vi "State.vi"(8 "error in (no error)":errorcluster caption="entrée d'erreur (pas d'erreur)", 10 "State":T1(ring), 11 "Actor_EventStart en entrée":refnum<class "Actor_EventStart.lvclass">) -> (0 "error out":errorcluster caption="sortie d'erreur", 3 "Actor_EventStart en sortie":refnum<class "Actor_EventStart.lvclass">)   [LabVIEW 2020, in "Library Core.lvlib" / "Actor_EventStart.lvlib" / "Actor_EventStart.lvclass"]
uses:
  Actor_EventStart.lvclass
  Commun VI/TypeDef/Variable Printable.ctl
  Actor_EventStart.lvclass/Actor_EventStart.ctl
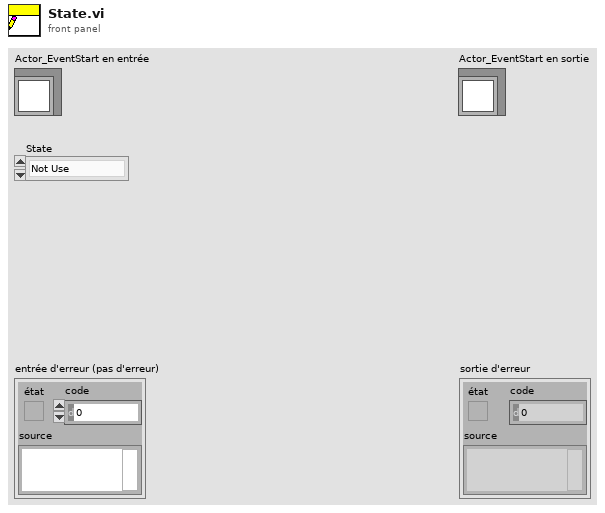
[diagram p1: front panel]
types:
  T1 = enum16{"Not Use", "Wait Event", "Test in progress", "Test Stopped"}
  T2 = enum16{"Get Variable", "Get All Variables", "Set Variable", "Delete Variable", "Delete All Variable"}
  T3 = typedef "Variable Printable.ctl" = string
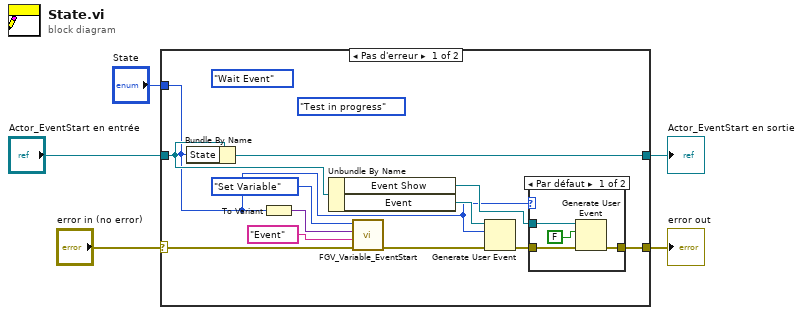
[diagram p0: block diagram]
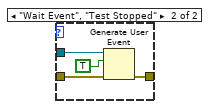
[diagram p2: hidden frame]
diagram:
  n1 = case shown="Pas d'erreur" "error in (no error)" {
    selector: "error in (no error)" -> [w9 w26]
    tunnel: [w15 w26] -> w4
    tunnel: [w17 w27] -> w2
    tunnel: "Actor_EventStart en entrée" -> [w16 w27]
    tunnel: "State" -> [w7 _]
    frame No Error {
      (unwired) T1."Wait Event" ("données d'événement")
      (unwired) T1."Test in progress" ("State")
      n2 = Bundle By Name(cluster=w16, "State"=w7) -> (w17:refnum<class "Actor_EventStart.lvclass">)
      n3 = To Variant(anything=w7) -> (Variant=w6:variant)
      n4 = Unbundle By Name(w16) -> ("Event Show"=w14:refnum<user-event>, "Event"=w12:refnum<user-event>)
      n5 = call "FGV_Variable_EventStart.vi"("error in (no error)"=w9, "Variable"=T3 "Event", "Data In"=w6, "Function"=T2."Set Variable") -> ("error out"=w8:errorcluster)  [unwired: 5 in, 2 out]
      n6 = Generate User Event(user event=w12, event data cluster=w7, error in=w8) -> (error out=w13:errorcluster)  [unwired: 1 in, 1 out]
      n7 = case shown="Par défaut" w7 {
        tunnel: w13 -> [w21 w22]
        tunnel: [w20 w25] -> w15
        tunnel: w14 -> [w18 w24]
        frame Default {
          n8 = Generate User Event(user event=w18, event data cluster=FALSE ("données d'événement"), error in=w21) -> (error out=w20:errorcluster)  [unwired: 1 in, 1 out]
        }
        frame "Wait Event", "Test Stopped" {
          n9 = Generate User Event(user event=w24, event data cluster=TRUE ("event data"), error in=w22) -> (error out=w25:errorcluster)  [unwired: 1 in, 1 out]
        }
      }
    }
    frame Error {
    }
  }
  "error out" <- w4
  "Actor_EventStart en sortie" <- w2
